vi "Set Dependent File Properties.vi"(7 "Format Settings":T2, 8 "error in (no error)":errorcluster, 10 "Dependent Files":T3[](array[typedef]), 11 "Device Ref in":T1 format="%.0x") -> (0 "error out":errorcluster, 3 "Device Ref out":T1 format="%.0x")   [LabVIEW 2019, in "SEECD System Explorer.lvlib"]
uses:
  <vilib>/NI VeriStand/Custom Device API/Custom Device File Dependency.ctl
  <vilib>/NI VeriStand/Custom Device API/Path Specification.ctl
  <vilib>/NI VeriStand/Custom Device API/Path Type.ctl
  <vilib>/NI VeriStand/Custom Device API/Custom Device Supported Target.ctl
  <vilib>/NI VeriStand/Custom Device API/Custom Device Item Ref.ctl
  NationalInstruments.VeriStand.SystemDefinitionAPI
  NationalInstruments.VeriStand.SystemStorage
  SEECD System Explorer.lvlib
  <vilib>/NI VeriStand/Custom Device API/Custom Device API.lvlib
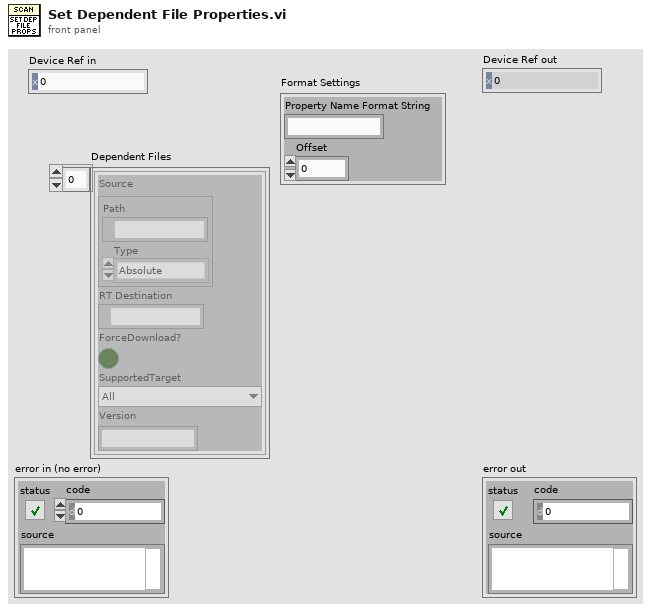
[diagram p1: front panel]
types:
  T1 = typedef "Custom Device API.lvlib/Custom Device Item Ref.ctl" = u64
  T2 = cluster{"Property Name Format String":string, "Offset":i32}
  T3 = typedef "Custom Device API.lvlib/Custom Device File Dependency.ctl" = cluster{"Source":T4, "RT Destination":path, "ForceDownload?":bool, "SupportedTarget":T6, "Version":string}
  T4 = typedef "Custom Device API.lvlib/Path Specification.ctl" = cluster{"Path":path, "Type":T5}
  T5 = typedef "Custom Device API.lvlib/Path Type.ctl" = enum16{"Absolute", "To Base", "To Common Data Dir", "To Application Data Dir"}
  T6 = typedef "Custom Device API.lvlib/Custom Device Supported Target.ctl" = enum16{"All", "PharLap", "VxWorks", "Windows", "Linux_32_ARM", "Linux_x64", "PharLap & Windows", "PharLap & VxWorks", "VxWorks & Windows"}
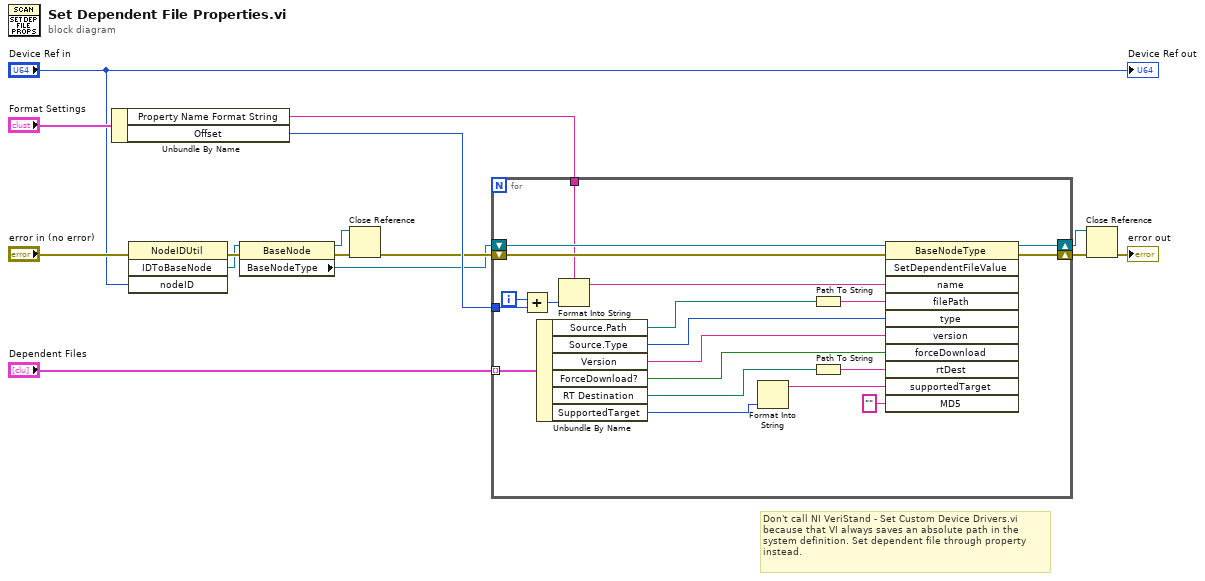
[diagram p0: block diagram]
diagram:
  # "Don't call NI VeriStand - Set Custom Device Drivers.vi\nbecause that VI always saves an absolute path in the\nsystem definition. Set dependent file through property\ninstead."
  n1 = Unbundle By Name("Format Settings") -> ("Property Name Format String"=w13:string, "Offset"=w12:i32)
  n2 = invoke class="NodeIDUtil" method="IDToBaseNode"(error in="error in (no error)", "nodeID"="Device Ref in") -> (error out=w9:errorcluster, "IDToBaseNode"=w8:refnum<k24>)  [unwired: 2 in, 2 out]
  n3 = property class="BaseNode"(reference=w8, error in=w9) -> (reference out=w7:refnum<k24>, error out=w10:errorcluster, "BaseNodeType"=w4:refnum<k24>)
  n4 = Close Reference(reference=w7, error in (no error)=w10) -> (error out=w5:errorcluster)
  n5 = for {
    shift-right: [w32] -> w15
    shift-left: w5 -> [w35]
    shift-right: [w33] -> w2
    shift-left: w4 -> [w34]
    tunnel: "Dependent Files" -> [w31] mode=indexing
    tunnel: w13 -> [w22]
    tunnel: w12 -> [w19]
    i -> [w21]
    n6 = Add(x=w21, y=w19) -> (x+y=w20:i32)
    n7 = Unbundle By Name(w31) -> ("Source.Path"=w29:path, "Source.Type"=w28:T5, "Version"=w27:string, "ForceDownload?"=w16:bool, "RT Destination"=w26:path, "SupportedTarget"=w24:T6)
    n8 = Format Into String(format string=w22, w20) -> (resulting string=w30:string)  [unwired: 2 in, 1 out]
    n9 = Format Into String(w24) -> (resulting string=w23:string)  [unwired: 3 in, 1 out]
    n10 = Path To String(path=w29) -> (string=w17:string)
    n11 = Path To String(path=w26) -> (string=w18:string)
    n12 = invoke class="BaseNodeType" method="SetDependentFileValue"(reference=w34, error in=w35, "name"=w30, "filePath"=w17, "type"=w28, "version"=w27, "forceDownload"=w16, "rtDest"=w18, "supportedTarget"=w23, "MD5"="") -> (reference out=w33:refnum<k24>, error out=w32:errorcluster)  [unwired: 1 in, 9 out]
  }
  n13 = Close Reference(reference=w2, error in (no error)=w15) -> (error out=→"error out":errorcluster)
  "Device Ref out" <- "Device Ref in"
